vi "niFPGA I32xI32 Dot Product - 3 elements I64.vi"(0 "A[I32]":i32[](array[numeric])=[0, 0, 0], 5 "B[I32]":i32[](array[numeric])=[0, 0, 0]) -> (7 "A.B [I64]":i64=2838)   [LabVIEW 2017]
uses:
  <vilib>/Platform/TimedLoop/XDataNode/timing_clust.ctl
  <vilib>/Platform/TimedLoop/XDataNode/nitl_modes.ctl
  <vilib>/Platform/TimedLoop/XDataNode/wakeup.ctl
  <vilib>/Platform/TimedLoop/XDataNode/XDataNode.xnode
  <vilib>/Platform/TimedLoop/XDataNode/XDNodeRunTimeDep.lvlib
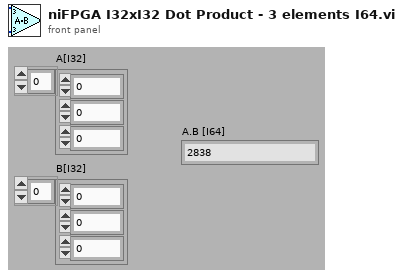
[diagram p1: front panel]
types:
  T1 = typedef "XDNodeRunTimeDep.lvlib/timing_clust.ctl" = cluster{"Expected End [f-1]":u64, "Actual End [f-1]":u64, "Finished Late? [f-1]":bool, "Expected End [i-1]":u64, "Actual End [i-1]":u64, "Finished Late? [i-1]":bool, "Expected Start [i]":u64, "Actual Start [i]":u64, "Expected Start [f]":u64, "Actual Start [f]":u64, "Source Name":string, "Structure Name":string, "Period":i64, "Deadline":i64, "Offset":i64, "Start":i64, "Priority":i32, "Timeout":i32, "Mode":T2, "Wakeup Reason":T3, "Error":errorcluster, "Source Type":string, "Secondary Source Type":string, "Global End Time":u64, "Global Start Time":u64, "Frame Duration":u64, "Iteration Duration":u64, "Assigned CPU":i32, "I/O Scan Engine Mode":u32}
  T2 = typedef "XDNodeRunTimeDep.lvlib/nitl_modes.ctl" = enum32{"No Change", "Process missed periods, maintain original phase", "Discard missed periods, maintain original phase", "Process missed periods, ignore original phase", "Discard missed periods, ignore original phase"}
  T3 = typedef "XDNodeRunTimeDep.lvlib/wakeup.ctl" = enum32{"Normal", "Aborted", "Asynchronous wakeup", "Timing source error", "Timed loop error", "Timeout"}
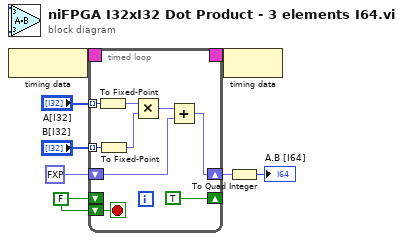
[diagram p0: block diagram]
diagram:
  w4 = FALSE
  n1 = node-c288() -> (w8:T1)
  n2 = timed-loop {
    shift-left: w4 -> [_]
    shift-right: [TRUE] -> _
    shift-left: fxp<+/-,64,64> 0.0 -> [w10]
    shift-right: [w9] -> w2
    tunnel: "A[I32]" -> [w11] mode=indexing
    tunnel: "B[I32]" -> [w12] mode=indexing
    timing: w8 -> [_]
    timing-out: [_] -> w7
    shift-left: w4 -> [w16]
    stop <- w16 stop-if-true
    n3 = To Fixed-Point(number=w11) -> (fixed-point=w14:fxp<+/-,32,32>)  [unwired: 1 out]
    n4 = To Fixed-Point(number=w12) -> (fixed-point=w13:fxp<+/-,32,32>)  [unwired: 1 out]
    n5 = Multiply(x=w14, y=w13) -> (x*y=w15:fxp<+/-,64,64>)
    n6 = Add(x=w15, y=w10) -> (x+y=w9:fxp<+/-,64,64>)
  }
  n7 = node-c288(w7) -> ()
  n8 = To Quad Integer(1:w2) -> (0:→"A.B [I64]":i64)
